vi "Analog oraz pomiar temp.vi"() -> ()   [LabVIEW 2014]
uses:
  Kontrolki/KartaDAQ/ACQ counter channel config.ctl
  Kontrolki/KartaDAQ/ACQ all read tasks.ctl
  Kontrolki/KartaDAQ/ACQ Params.ctl
  Kontrolki/KartaDAQ/ACQ analog channel config new.ctl
panel:
  out "dalta średnia":dbl
  out "Array of delays":dbl[](array[numeric])
  out "DevTemp":dbl
  out "delta":dbl
  in  "stop":bool
  out "Waveform Graph":waveform(dbl)[](graph)
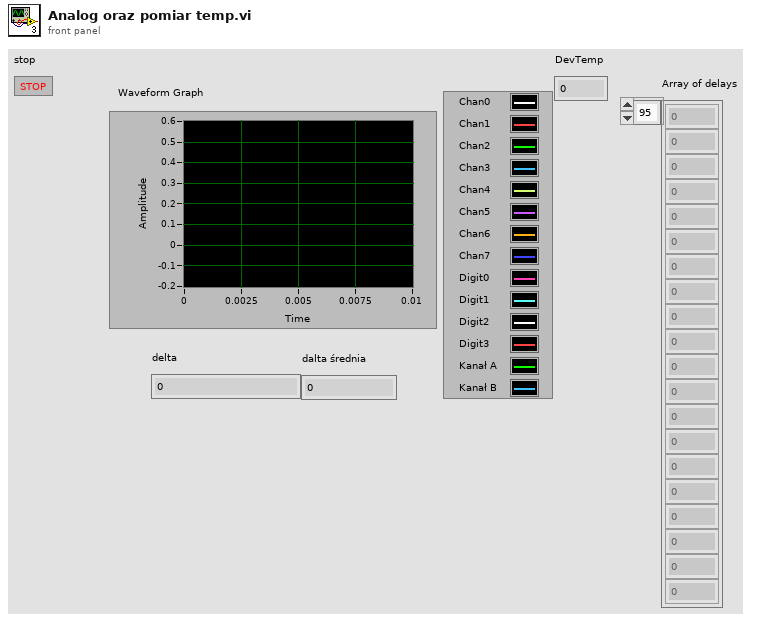
[diagram p1: front panel]
types:
  T1 = typedef "ACQ analog channel config new.ctl" = cluster{"Analogs IN":string[], "Digitals IN":string[]}
  T2 = typedef "ACQ Params.ctl" = cluster{"Analog":cluster{"minimum value":dbl, "maximum value":dbl}, "Digital":cluster{"minimum value":dbl, "maximum value":dbl}, "Time":cluster{"sample mode":i32, "samples per channel in":i32, "rate":dbl, "active edge":i32}, "AI common":cluster{"input terminal configuration":i32, "source":string}, "Enkoder":cluster{"channel1 name":string, "channel2 name":string, "units":i32, "initial position":dbl, "distance per pulse":dbl, "z index enable":bool, "z index value":dbl, "z index phase":i32, "decoding type":i32}}
  T3 = typedef "ACQ all read tasks.ctl" = cluster{"Analog ref":refnum<k21>, "Enkoder X ref":refnum<k21>, "Enkoder Y ref":refnum<k21>, "Generator ref":refnum<k21>}
  T4 = typedef "ACQ counter channel config.ctl" = cluster{"Enkoder X":string, "Enkoder Y":string, "Generator":string, "Generator OUT":string}
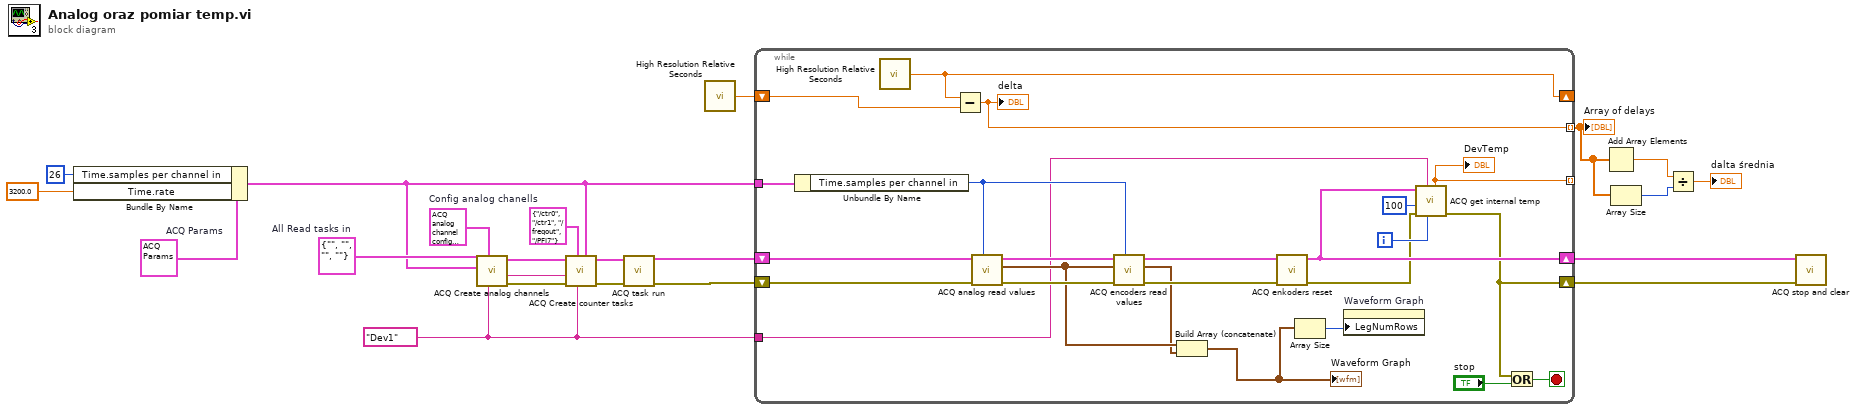
[diagram p0: block diagram]
diagram:
  w13 = T1 {"Analogs IN"=["/ai1", "/ai9", "/ai2", "/ai10", "/ai3", "/ai11", "/ai4", "/ai12"], "Digitals IN"=["/ai7", "/ai6", "/ai14", "/ai15"]}  # Config analog chanells
  w5 = tag "Dev1" ("device in")
  w20 = T2 {"Analog"={"minimum value"=-1.0, "maximum value"=1.0}, "Digital"={"minimum value"=0.0, "maximum value"=5.0}, "Time"={"sample mode"=10123, "samples per channel in"=26, "rate"=3200.0, "active edge"=10280}, "AI common"={"input terminal configuration"=10083, "source"="/ai/SampleClock"}, "Enkoder"={"channel1 name"="Linear X", "channel2 name"="Linear Y", "units"=10219, "initial position"=0.0, "distance per pulse"=1.0, "z index enable"=FALSE, "z index value"=0.0, "z index phase"=10040, "decoding type"=10091}}  # ACQ Params
  w12 = T3 {"Analog ref"="", "Enkoder X ref"="", "Enkoder Y ref"="", "Generator ref"=""}  # All Read tasks in
  n1 = Bundle By Name(cluster=w20, "Time.samples per channel in"=26, "Time.rate"=3200.0) -> (w7:T2)
  n2 = call "ACQ Create analog channels.vi"("device in"=w5, "Config analog chanells new"=w13, "ACQ Params"=w7, "All Read tasks in"=w12) -> ("error out"=w15:errorcluster, "Terminal Name with Device Prefix"=w14:tag, "All Read tasks out"=w19:T3)  [unwired: 4 in, 1 out]
  n3 = call "ACQ Create counter tasks.vi"("ACQ Params"=w7, "device in"=w5, "Config Counter channels"=T4 {"Enkoder X"="/ctr0", "Enkoder Y"="/ctr1", "Generator"="/freqout", "Generator OUT"="/PFI7"}, "error in (no error)"=w15, "Terminal Name with Device Prefix"=w14, "All Read tasks in"=w19) -> ("error out"=w16:errorcluster, "All Read tasks out"=w17:T3)  [unwired: 4 in]
  n4 = call "ACQ task run.vi"("error in (no error)"=w16, "All Read tasks in"=w17) -> ("error out"=w11:errorcluster, "All Read tasks out"=w10:T3)  [unwired: 7 in, 1 out]
  n5 = call <vilib>:"High Resolution Relative Seconds.vi"() -> ("relative seconds"=w6:dbl)
  n6 = while {
    tunnel: w7 -> [w40]
    shift-right: [w23] -> w9
    shift-left: w11 -> [w46]
    shift-right: [w31] -> w8
    shift-left: w10 -> [w45]
    shift-right: [w34] -> _
    shift-left: w6 -> [w33]
    tunnel: w5 -> [w30]
    tunnel: [w28] -> w4 mode=indexing
    tunnel: [w27] -> _ mode=indexing
    i -> [w32]
    stop <- w24 stop-if-true
    n7 = Unbundle By Name(w40) -> ("Time.samples per channel in"=w39:i32)
    n8 = call <vilib>:"High Resolution Relative Seconds.vi"() -> ("relative seconds"=w34:dbl)
    n9 = Subtract(x=w34, y=w33) -> (x-y=w28:dbl)
    "delta" <- w28
    n10 = call "ACQ analog read values.vi"("samples per channel"=w39, "error in (no error)"=w46, "Tasks ref in"=w45) -> ("error out"=w44:errorcluster, "data"=w37:waveform(dbl)[], "Tasks ref out"=w43:T3)  [unwired: 6 in]
    n11 = call "ACQ encoders read values.vi"("samples per channel"=w39, "error in (no error)"=w44, "AI data"=w37, "Tasks ref in"=w43) -> ("error out"=w42:errorcluster, "Enk wfm out"=w35:waveform(dbl)[], "Tasks ref out"=w41:T3)  [unwired: 5 in]
    n12 = Build Array (concatenate)(w37, w35) -> (w36:waveform(dbl)[])
    "Waveform Graph" <- w36
    n13 = call "ACQ enkoders reset.vi"("error in (no error)"=w42, "Tasks ref in"=w41) -> ("error out"=w26:errorcluster, "Tasks ref out"=w31:T3)  [unwired: 8 in]
    n14 = Array Size(array=w36) -> (size(s)=w38:i32)
    n15 = property on="Waveform Graph" class="WFGraph (strict)"("LegNumRows"=w38) -> ()  [unwired: 2 in, 2 out]
    n16 = call "ACQ get internal temp.vi"("i"=w32, "Urządzenie"=w30, "error in (no error)"=w26, "div (300)"=100, "Tasks ref in"=w31) -> ("error out"=w23:errorcluster, "DevTemp"=w27:dbl)  [unwired: 4 in, 1 out]
    "DevTemp" <- w27
    n17 = Or(x=w23, y="stop") -> (x .or. y?=w24:bool)
  }
  "Array of delays" <- w4
  n18 = Add Array Elements(numeric array=w4) -> (sum=w3:dbl)
  n19 = Array Size(array=w4) -> (size(s)=w2:i32)
  n20 = Divide(x=w3, y=w2) -> (x/y=→"dalta średnia":dbl)
  n21 = call "ACQ stop and clear.vi"("error in (no error)"=w9, "Tasks ref in"=w8) -> ()  [unwired: 9 in, 1 out]
